vi "Debug - Close.vi"(8 "error in (no error)":errorcluster, 11 "Debug Resources":T1) -> (0 "error out":errorcluster)   [LabVIEW 2021, in "UDP-Custom-Device Engine.lvlib"]
uses:
  UDP-Custom-Device Engine.lvlib
  Types/Engine - Debug Resources.ctl
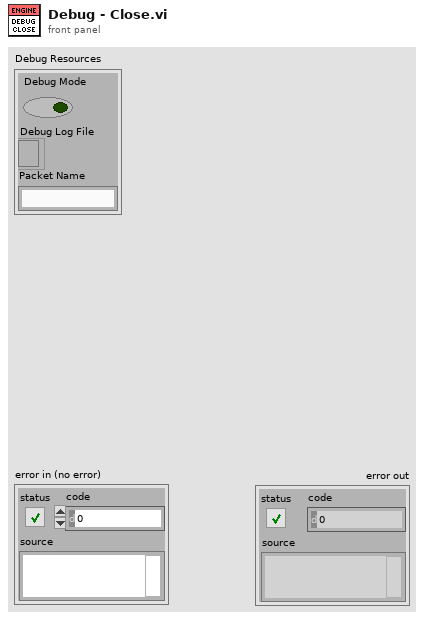
[diagram p1: front panel]
types:
  T1 = typedef "UDP-Custom-Device Engine.lvlib/Engine - Debug Resources.ctl" = cluster{"Debug Mode":bool, "Debug Log File":refnum<file>, "Packet Name":string}
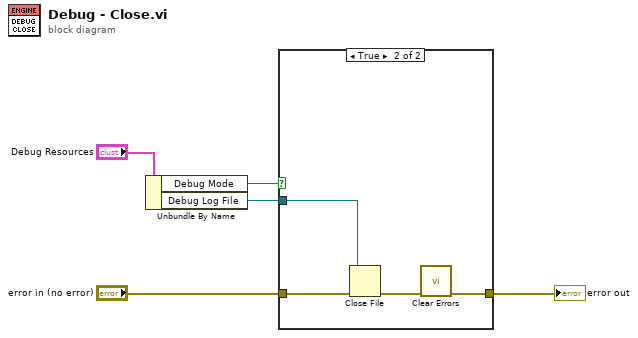
[diagram p0: block diagram]
diagram:
  n1 = Unbundle By Name("Debug Resources") -> ("Debug Mode"=w2:bool, "Debug Log File"=w1:refnum<file>)
  n2 = case shown="True" w2 {
    tunnel: "error in (no error)" -> [w6 w9]
    tunnel: [w6 w7] -> w4
    tunnel: w1 -> [_ w10]
    frame False {
    }
    frame True {
      n3 = Close File(refnum=w10, error in=w9) -> (error out=w8:errorcluster)  [unwired: 1 out]
      n4 = call <vilib>:"Clear Errors.vi"("error in (no error)"=w8) -> ("error out"=w7:errorcluster)  [unwired: 5 in, 1 out]
    }
  }
  "error out" <- w4
